vi "Set Framed Project Path.vi"(8 "error in (no error)":errorcluster, 10 "Framed Project Path":path, 11 "Edit Project Model in":refnum<class "Edit Project Model.lvclass">) -> (0 "error out":errorcluster, 3 "Edit Project Model out":refnum<class "Edit Project Model.lvclass">)   [LabVIEW 2013, in "Edit Project Model.lvlib" / "Edit Project Model.lvclass"]
uses:
  Edit Project Model.lvclass
  Edit Project Model.lvclass/Edit Project Model.ctl
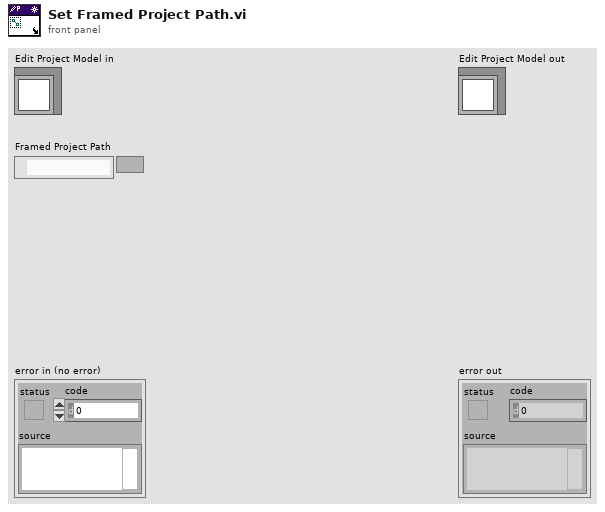
[diagram p1: front panel]
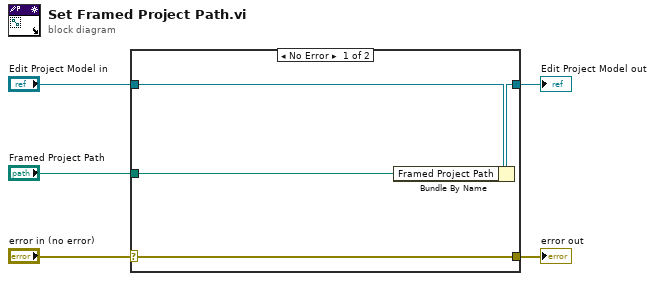
[diagram p0: block diagram]
diagram:
  n1 = case shown="No Error" "error in (no error)" {
    selector: "error in (no error)" -> [w9 w10]
    tunnel: [w9 w10] -> w4
    tunnel: [w7 w11] -> w2
    tunnel: "Edit Project Model in" -> [w8 w11]
    tunnel: "Framed Project Path" -> [w6 _]
    frame No Error {
      n2 = Bundle By Name(cluster=w8, "Framed Project Path"=w6) -> (w7:refnum<class "Edit Project Model.lvclass">)
    }
    frame Error {
    }
  }
  "error out" <- w4
  "Edit Project Model out" <- w2
